vi "Cleanup Session.vi"(8 "error in":errorcluster, 11 "Plugin in":refnum<class "Statistic.lvclass">) -> (0 "error out":errorcluster, 3 "Plugin out":refnum<class "Statistic.lvclass">)   [LabVIEW 2025, in "Statistic.lvlib" / "Statistic.lvclass"]
uses:
  Statistic.lvclass
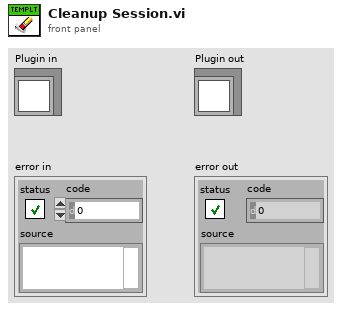
[diagram p1: front panel]
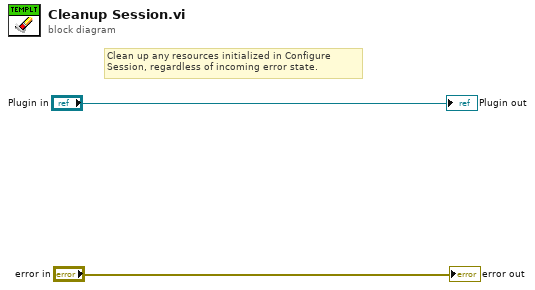
[diagram p0: block diagram]
diagram:
  # "Clean up any resources initialized in Configure Session, regardless of incoming error state."
  "error out" <- "error in"
  "Plugin out" <- "Plugin in"
